vi "全局 数据发送重叠.vi"() -> ()   [LabVIEW 2016, in "数据传输系统-03.lvlib"]
panel:
  out "数据接收超时指示灯":bool
  out "主动上报数据中":bool
  in  "TCP掉线时间节点":string
  in  "掉线指示灯":bool
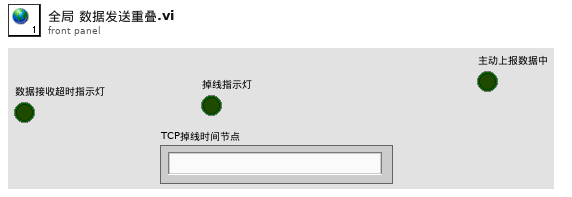
[diagram p1: front panel]
diagram:
